vi "Parallel Data Read Example.vi"() -> ()   [LabVIEW 2018]
uses:
  NiFpga.dll
panel:
  out "SGL":sgl
  out "U16":u16
  out "I8":i8
  out "U8":u8
  out "Waveform Graph":dbl[](graph)
  out "Average":dbl
  out "FXP Value":dbl
  out "error out":errorcluster
  in  "Error In":errorcluster
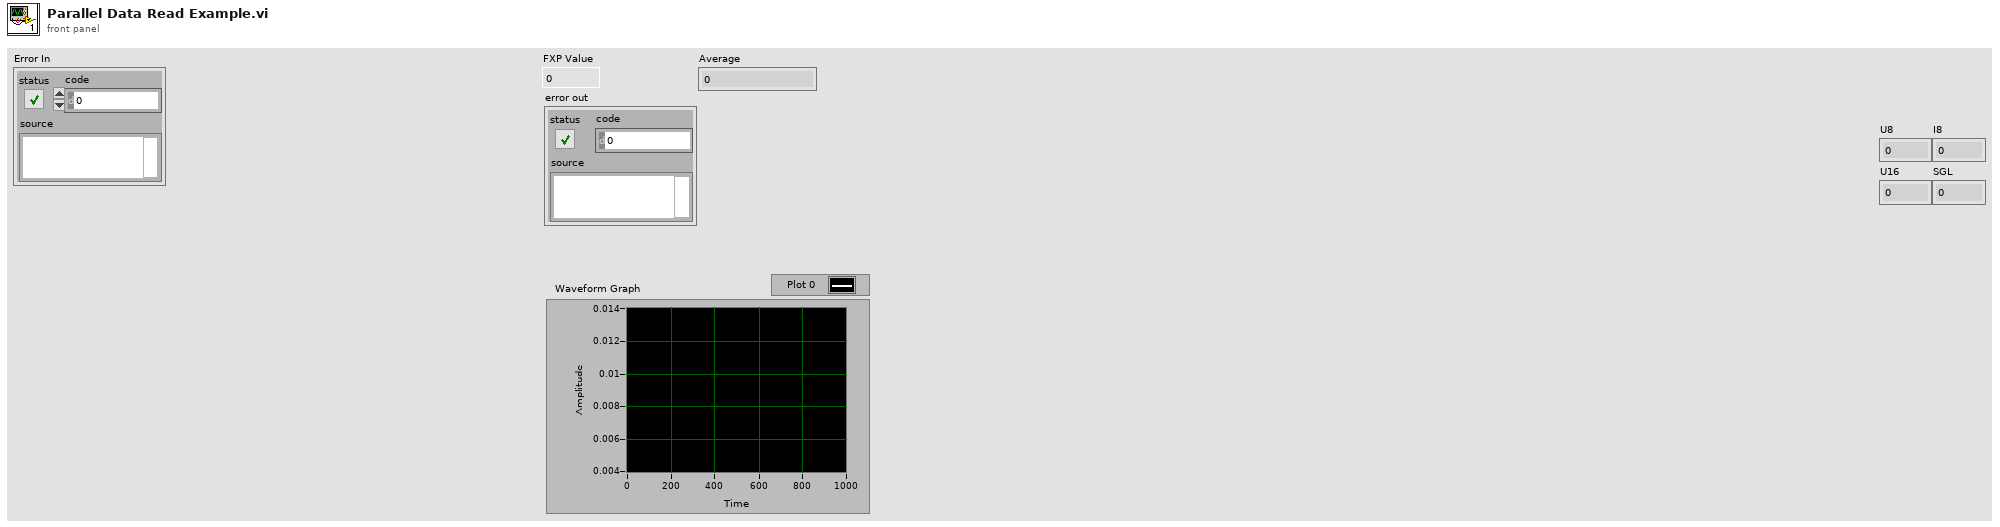
[diagram p1: front panel]
types:
  T1 = cluster{"Delta":dbl, "Word Length":i8, "Signed":bool, "offset":i32, "Name":string, "base address":i32}[]
  T2 = cluster{"Delta":dbl, "Word Length":i8, "Signed":bool, "offset":i32, "Name":string, "base address":i32}
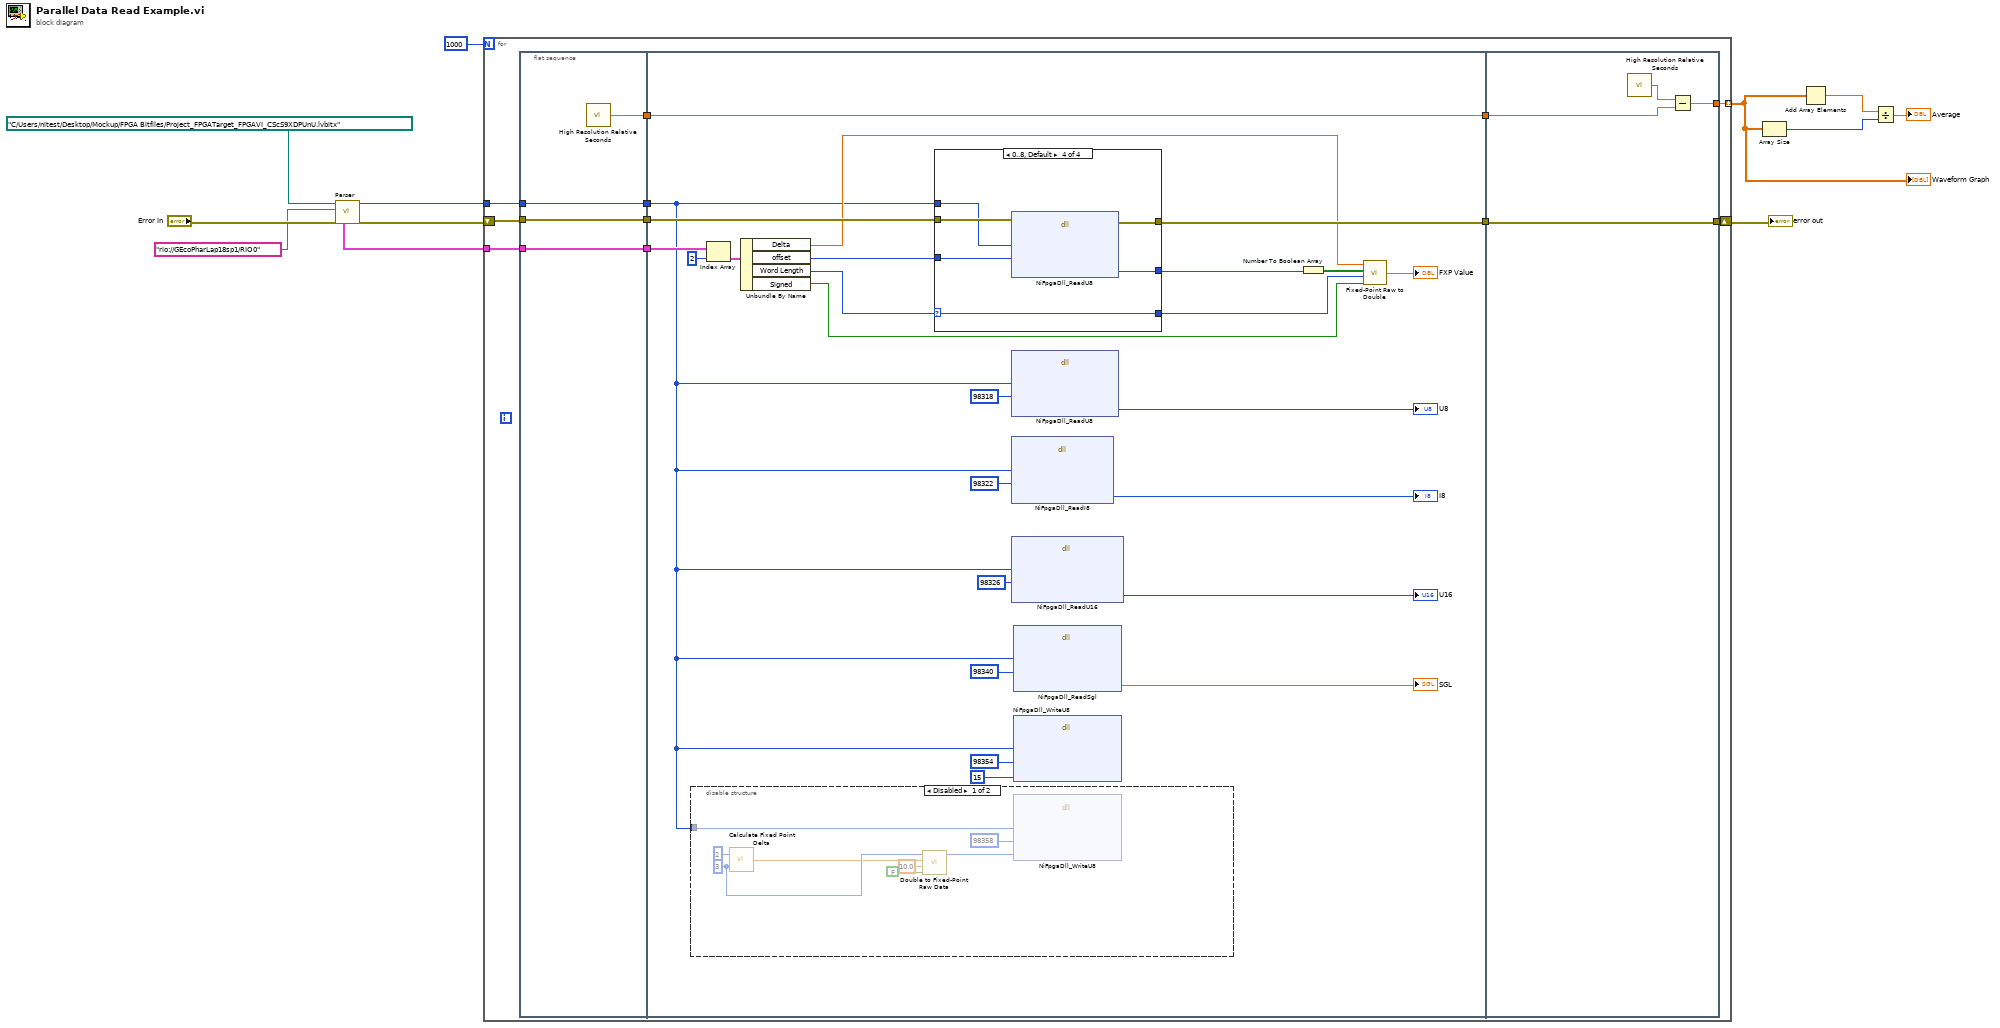
[diagram p0: block diagram]
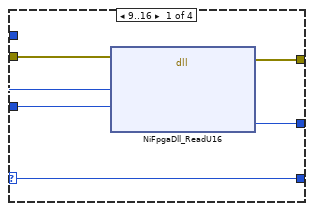
[diagram p3: hidden frame]
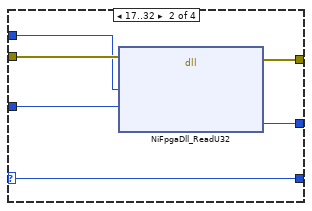
[diagram p4: hidden frame]
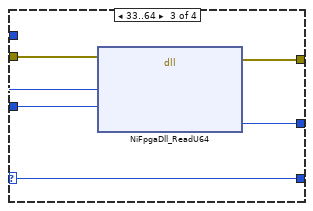
[diagram p5: hidden frame]
diagram:
  n1 = call "Parser.vi"("error in (no error)"="Error In", "RIO device address"="rio://GEcoPharLap18sp1/RIO0" ("Device address"), "bitfile path"=path "C:/Users/nitest/Desktop/Mockup/FPGA Bitfiles/Project_FPGATarget_FPGAVI_CScS9XDPUnU.lvbitx" ("Bitfile path")) -> ("error out"=w9:errorcluster, "FXP channels out"=w6:T1, "session out"=w7:u64)  [unwired: 6 in]
  n2 = for {
    N: 1000 -> [_]
    tunnel: w7 -> [w21]
    tunnel: w6 -> [w20]
    shift-right: [w23] -> w12
    shift-left: w9 -> [w22]
    tunnel: [w13] -> w1 mode=indexing
    n3 = flat-sequence {
      tunnel: w20 -> [w25]
      tunnel: w21 -> [w26]
      tunnel: w22 -> [w27]
      tunnel: [w27] -> w19
      tunnel: [w26] -> w18
      tunnel: [w25] -> w17
      tunnel: [w24] -> w14
      tunnel: w19 -> [w47]
      tunnel: w18 -> [w28]
      tunnel: w17 -> [w46]
      tunnel: [w52] -> w16
      tunnel: [w39] -> w15
      tunnel: w14 -> [w39]
      tunnel: [w88] -> w23
      tunnel: w16 -> [w88]
      tunnel: w15 -> [w86]
      tunnel: [w85] -> w13
      frame #0 {
        n4 = call <vilib>:"High Resolution Relative Seconds.vi"() -> ("relative seconds"=w24:dbl)
      }
      frame #1 {
        n5 = disable-structure shown="Disabled" {
          disable-tunnel: w28 -> [w60 _]
          frame Disabled {
            w57 = u8 3 ("WordLength")
            n6 = call "Calculate Fixed Point Delta.vi"("WordLength"=w57, "IntegerWordLength"=2) -> ("delta"=w56:dbl)
            n7 = call "Double to Fixed-Point Raw Data.vi"("isSigned?"=FALSE, "data"=sgl 10.0, "delta"=w56, "word length"=w57) -> ("Value"=w53:i64)  [unwired: 7 in]
            n8 = dll-call lib="NiFpga.*" fn="NiFpgaDll_WriteU8"("session"=w60, "control"=u32 98358, "value"=w53) -> ()  [unwired: 7 in, 2 out]
          }
          frame Enabled {
          }
        }
        n9 = Index Array(array=w46, index=2) -> (element=w44:T2)
        n10 = Unbundle By Name(w44) -> ("Delta"=w40:dbl, "offset"=w43:i32, "Word Length"=w42:i8, "Signed"=w41:bool)
        n11 = case shown="0..8, Default" w42 {
          selector: w42 -> [w64 w70 w76 w82]
          tunnel: [w66 w71 w78 w84] -> w52
          tunnel: [w65 w72 w77 w83] -> w51
          tunnel: [w64 w70 w76 w82] -> w48
          tunnel: w47 -> [w63 w69 w75 w81]
          tunnel: w28 -> [w61 w67 w74 w80]
          tunnel: w43 -> [w62 w68 w73 w79]
          frame 9..16 {
            n12 = dll-call lib="NiFpga.*" fn="NiFpgaDll_ReadU16"(error in=w63, "session"=w61, "offset"=w62) -> (error out=w66:errorcluster, "value"=w65:u8)  [unwired: 6 in, 1 out]
          }
          frame 17..32 {
            n13 = dll-call lib="NiFpga.*" fn="NiFpgaDll_ReadU32"(error in=w69, "session"=w67, "offset"=w68) -> (error out=w71:errorcluster, "value"=w72:u8)  [unwired: 6 in, 1 out]
          }
          frame 33..64 {
            n14 = dll-call lib="NiFpga.*" fn="NiFpgaDll_ReadU64"(error in=w75, "session"=w74, "offset"=w73) -> (error out=w78:errorcluster, "value"=w77:u8)  [unwired: 6 in, 1 out]
          }
          frame 0..8, Default {
            n15 = dll-call lib="NiFpga.*" fn="NiFpgaDll_ReadU8"(error in=w81, "session"=w80, "offset"=w79) -> (error out=w84:errorcluster, "value"=w83:u8)  [unwired: 6 in, 1 out]
          }
        }
        n16 = dll-call lib="NiFpga.*" fn="NiFpgaDll_ReadU8"("session"=w28, "offset"=u32 98318) -> ("value"=→"U8":u8)  [unwired: 7 in, 2 out]
        n17 = dll-call lib="NiFpga.*" fn="NiFpgaDll_ReadI8"("session"=w28, "offset"=u32 98322) -> ("value"=→"I8":i8)  [unwired: 7 in, 2 out]
        n18 = dll-call lib="NiFpga.*" fn="NiFpgaDll_ReadU16"("session"=w28, "offset"=u32 98326) -> ("value"=→"U16":u16)  [unwired: 7 in, 2 out]
        n19 = dll-call lib="NiFpga.*" fn="NiFpgaDll_ReadSgl"("session"=w28, "offset"=u32 98340 ("session")) -> ("value"=→"SGL":sgl)  [unwired: 7 in, 2 out]
        n20 = dll-call lib="NiFpga.*" fn="NiFpgaDll_WriteU8"("session"=w28, "control"=u32 98354, "value"=i8 15) -> ()  [unwired: 7 in, 2 out]
        n21 = Number To Boolean Array(number=w51) -> (Boolean array=w50:bool[])
        n22 = call "Fixed-Point Raw to Double.vi"("Signed?"=w41, "Word Length"=w48, "Data"=w50, "Delta"=w40) -> ("value"=→"FXP Value":dbl)
      }
      frame #2 {
        n23 = call <vilib>:"High Resolution Relative Seconds.vi"() -> ("relative seconds"=w87:dbl)
        n24 = Subtract(x=w87, y=w86) -> (x-y=w85:dbl)
      }
    }
  }
  "error out" <- w12
  "Waveform Graph" <- w1
  n25 = Array Size(array=w1) -> (size(s)=w3:i32)
  n26 = Add Array Elements(numeric array=w1) -> (sum=w4:dbl)
  n27 = Divide(x=w4, y=w3) -> (x/y=→"Average":dbl)
